vi "系统全局.vi"() -> ()   [LabVIEW 2014]
panel:
  out "告警状态":bool
  out "告警信息":string
  out "接收缓冲":string
  out "接收状态":bool
  out "串口状态":bool
  out "退出程序":bool
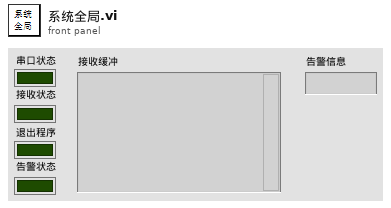
[diagram p1: front panel]
diagram:
